vi "Digital_Output_16Channels.vi"(1 "States":bool[](array[boolean])=[FALSE, FALSE, FALSE, FALSE, FALSE, FALSE, FALSE, FALSE, FALSE, FALSE, FALSE, FALSE, FALSE, FALSE, FALSE, FALSE], 2 "IO":T1={"DO 0"="Mod1/DIO2", "DO 1"="Mod1/DIO2", "DO 2"="Mod1/DIO2", "DO 3"="Mod1/DIO2", "DO 4"="Mod1/DIO2", "DO 5"="Mod1/DIO2", "DO 6"="Mod1/DIO2", "DO 7"="Mod1/DIO2", "DO 8"="Mod1/DIO2", "DO 9"="Mod1/DIO2", "DO 10"="Mod1/DIO2", "DO 11"="Mod1/DIO2", "DO 12"="Mod1/DIO2", "DO 13"="Mod1/DIO2", "DO 14"="Mod1/DIO2", "DO 15"="Mod1/DIO2"}) -> ()   [LabVIEW 2015, in "FPGA Wizard Templates.lvlib"]
uses:
  FPGA Wizard Templates.lvlib
  <vilib>/rvi/eio/common/nirviEmuTemplateMethod_errors.vi
  <vilib>/eio/EIONode/EIONode.xnode
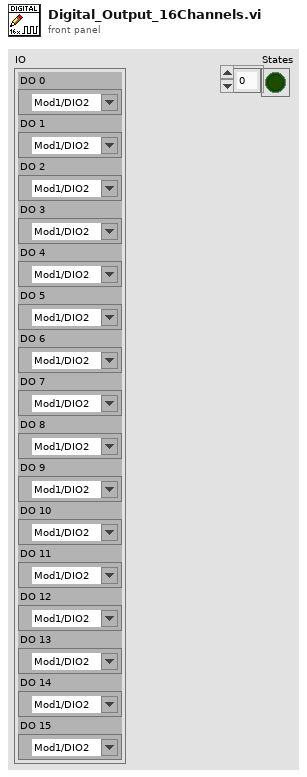
[diagram p1: front panel]
types:
  T1 = cluster{"DO 0":refnum<k21>, "DO 1":refnum<k21>, "DO 2":refnum<k21>, "DO 3":refnum<k21>, "DO 4":refnum<k21>, "DO 5":refnum<k21>, "DO 6":refnum<k21>, "DO 7":refnum<k21>, "DO 8":refnum<k21>, "DO 9":refnum<k21>, "DO 10":refnum<k21>, "DO 11":refnum<k21>, "DO 12":refnum<k21>, "DO 13":refnum<k21>, "DO 14":refnum<k21>, "DO 15":refnum<k21>}
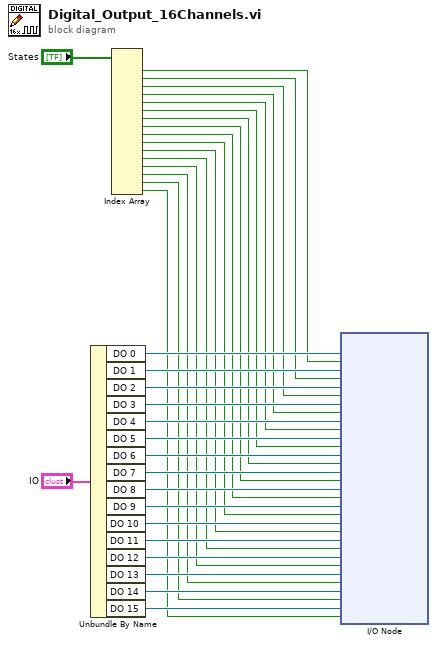
[diagram p0: block diagram]
diagram:
  n1 = Unbundle By Name("IO") -> ("DO 0"=w33:refnum<k21>, "DO 1"=w32:refnum<k21>, "DO 2"=w31:refnum<k21>, "DO 3"=w30:refnum<k21>, "DO 4"=w29:refnum<k21>, "DO 5"=w28:refnum<k21>, "DO 6"=w27:refnum<k21>, "DO 7"=w26:refnum<k21>, "DO 8"=w16:refnum<k21>, "DO 9"=w15:refnum<k21>, "DO 10"=w14:refnum<k21>, "DO 11"=w13:refnum<k21>, "DO 12"=w12:refnum<k21>, "DO 13"=w11:refnum<k21>, "DO 14"=w10:refnum<k21>, "DO 15"=w9:refnum<k21>)
  n2 = Index Array(array="States") -> (element #1=w24:bool, element #2=w23:bool, element #3=w22:bool, element #4=w21:bool, element #5=w20:bool, element #6=w19:bool, element #7=w18:bool, element #8=w17:bool, element #9=w8:bool, element #10=w7:bool, element #11=w6:bool, element #12=w5:bool, element #13=w4:bool, element #14=w3:bool, element #15=w2:bool, element #16=w1:bool)  [unwired: 16 in]
  n3 = xnode "I/O Node"("I/O Item"=w24, "FPGA I/O In"=w33, "I/O Item"=w23, "FPGA I/O In"=w32, "I/O Item"=w22, "FPGA I/O In"=w31, "I/O Item"=w21, "FPGA I/O In"=w30, "I/O Item"=w20, "FPGA I/O In"=w29, "I/O Item"=w19, "FPGA I/O In"=w28, "I/O Item"=w18, "FPGA I/O In"=w27, "I/O Item"=w17, "FPGA I/O In"=w26, "I/O Item"=w8, "FPGA I/O In"=w16, "I/O Item"=w7, "FPGA I/O In"=w15, "I/O Item"=w6, "FPGA I/O In"=w14, "I/O Item"=w5, "FPGA I/O In"=w13, "I/O Item"=w4, "FPGA I/O In"=w12, "I/O Item"=w3, "FPGA I/O In"=w11, "I/O Item"=w2, "FPGA I/O In"=w10, "I/O Item"=w1, "FPGA I/O In"=w9) -> ()  [unwired: 16 out]
